vi "jpg to pic.vi"(8 "error in (no error)":errorcluster, 11 "path to JPEG file":path) -> (0 "error out":errorcluster, 1 "Resized Picture":picture)   [LabVIEW 2017]
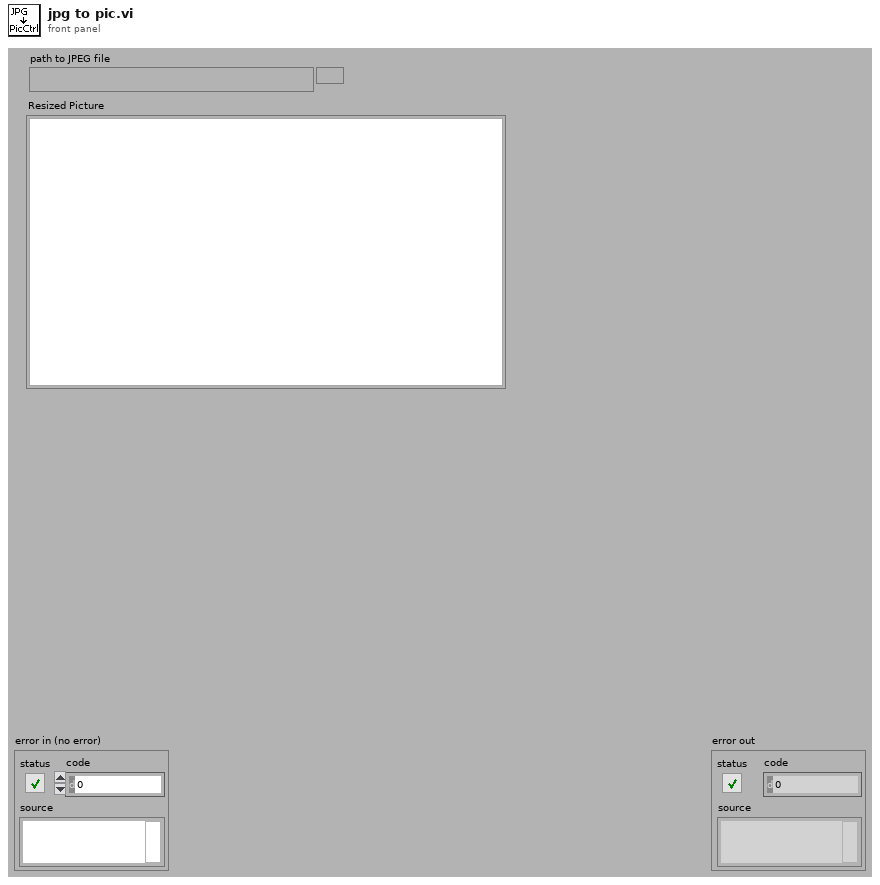
[diagram p1: front panel]
types:
  T1 = typedef "imagedata.ctl" = cluster{"image type":i32, "image depth":i32, "image":u8[], "mask":u8[], "colors":u32[], "Rectangle":cluster{"left":i16, "top":i16, "right":i16, "bottom":i16}}
  T2 = typedef "LVBoundsTypeDef.ctl" = cluster{"Width":u32, "Height":u32}
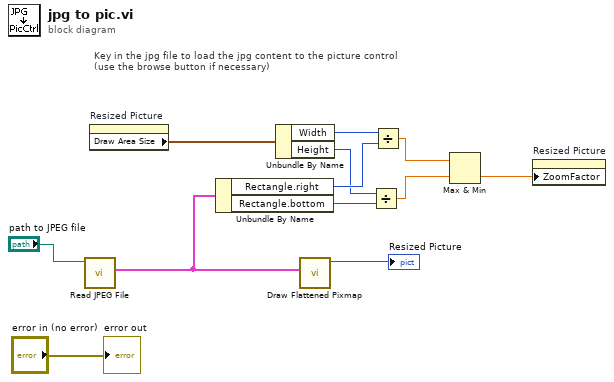
[diagram p0: block diagram]
diagram:
  # "Key in the jpg file to load the jpg content to the picture control\n(use the browse button if necessary)"
  n1 = call <vilib>:"Read JPEG File.vi"("path to JPEG file"="path to JPEG file") -> ("image data"=w9:T1)  [unwired: 8 in, 2 out]
  n2 = property on="Resized Picture" class="Pict"() -> ("Draw Area Size"=w8:T2)  [unwired: 2 in, 2 out]
  n3 = Unbundle By Name(w9) -> ("Rectangle.right"=w6:i16, "Rectangle.bottom"=w4:i16)
  n4 = Unbundle By Name(w8) -> ("Width"=w7:u32, "Height"=w5:u32)
  n5 = call <vilib>:"Draw Flattened Pixmap.vi"("image data"=w9) -> ("new picture"=→"Resized Picture":picture)  [unwired: 8 in]
  n6 = Divide(x=w5, y=w4) -> (x/y=w2:dbl)
  n7 = Divide(x=w7, y=w6) -> (x/y=w3:dbl)
  n8 = Max & Min(x=w3, y=w2) -> (min(x,y)=w1:dbl)  [unwired: 1 out]
  n9 = property on="Resized Picture" class="Pict"("ZoomFactor"=w1) -> ()  [unwired: 2 in, 2 out]
  "error out" <- "error in (no error)"
